vi "broadcast_ping.vi"() -> ()   [LabVIEW 2022 SP3]
uses:
  Library/dxl_x64_c.lvlib
panel:
  out "dynamixel_comm_result":string
  in  "dynamixel_id_list":string[][](table)=[[""], [""]]
  in  "device_name":string="COM1"
  out "protocol_version":dbl=2.0
  out "port_num":i32
  in  "baud_rate":i32=57600
  # "/*******************************************************************************\n* Copyright (c) 2016, ROBOTIS CO., LTD.\n* All rights reserved.\n*\n* Redistribution and use in source and binary forms, with or without\n* modification, are permitted provided that the following conditions are met:\n*\n* * Redistributions of source code must retain the above copyright notice, this\n*   list of conditions and the following disclaimer.\n*\n* * Redistributions in binary form must reproduce the above copyright notice,\n*   this list of conditions and the following disclaimer in the documentation\n*   and/or other materials provided with the distribution.\n*\n* * Neither the name of ROBOTIS nor the names of its\n*   contributors may be used to endorse or promote products derived from\n*   this software without specific prior written permission.\n*\n* THIS SOFTWARE IS PROVIDED BY THE COPYRIGHT HOLDERS AND CONTRIBUTORS \"AS IS\"\n* AND ANY EXPRESS OR IMPLIED WARRANTIES, INCLUDING, BUT NOT LIMITED TO, THE\n* IMPLIED WARRANTIES OF MERCHANTABILITY AND FITNESS FOR A PARTICULAR PURPOSE ARE\n* DISCLAIMED. IN NO EVENT SHALL THE COPYRIGHT HOLDER OR CONTRIBUTORS BE LIABLE\n* FOR ANY DIRECT, INDIRECT, INCIDENTAL, SPECIAL, EXEMPLARY, OR CONSEQUENTIAL\n* DAMAGES (INCLUDING, BUT NOT LIMITED TO, PROCUREMENT OF SUBSTITUTE GOODS OR\n* SERVICES; LOSS OF USE, DATA, OR PROFITS; OR BUSINESS INTERRUPTION) HOWEVER\n* CAUSED AND ON ANY THEORY OF LIABILITY, WHETHER IN CONTRACT, STRICT LIABILITY,\n* OR TORT (INCLUDING NEGLIGENCE OR OTHERWISE) ARISING IN ANY WAY OUT OF THE USE\n* OF THIS SOFTWARE, EVEN IF ADVISED OF THE POSSIBILITY OF SUCH DAMAGE.\n*******************************************************************************/\n\n/* Author: Ryu Woon Jung (Leon) */"
  # "Available Dynamixel model on this example : All models using Protocol 2.0\nThis example is designed for using Dynamixel PRO 54-200s, and an USB2DYNAMIXEL.\nTo use another Dynamixel model, such as X series, see their details in E-Manual(support.robotis.com) \n   and edit \"numeric control\"s seen left with \"Edit Text\" tool.\nBe sure that Dynamixel PRO properties are already set as %% ID : 1 / Baudnum : 1 (Baudrate : 57600)\n\n1. Run example by click above \"Run\" button (below \"Edit\" menu).\n2. You may see the ID list of connected Dynamixels."
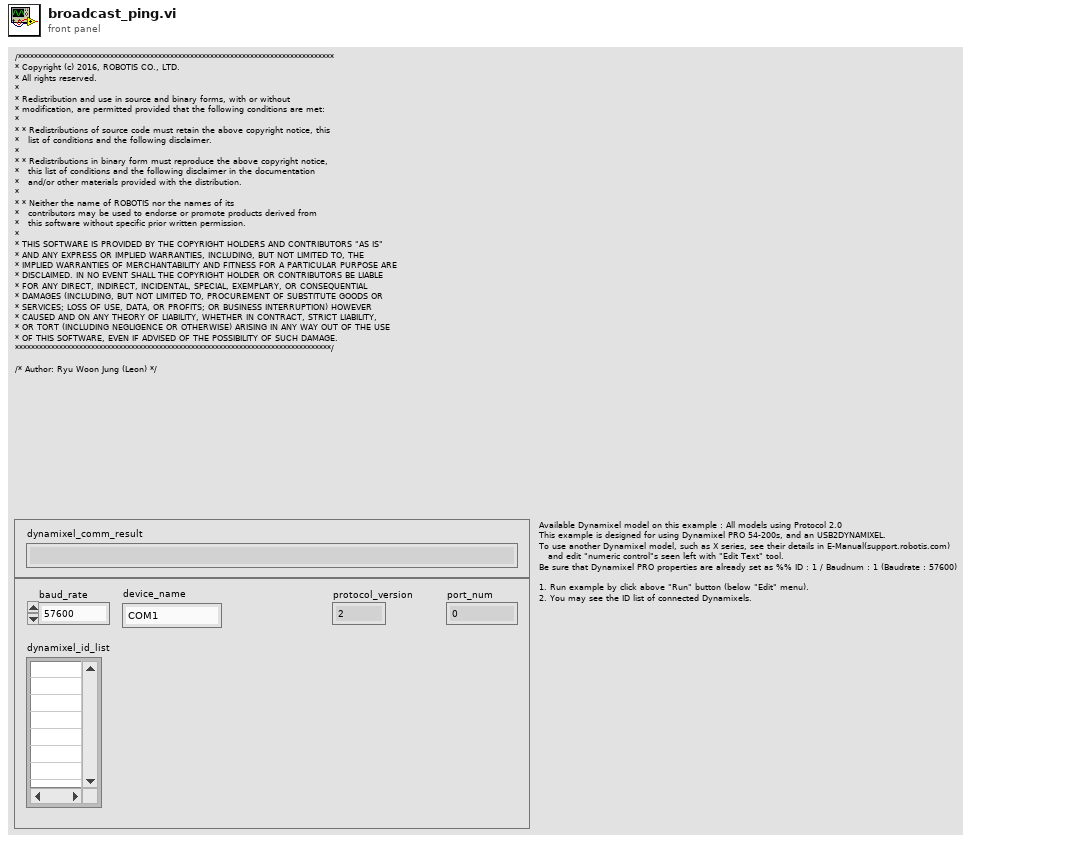
[diagram p1: front panel]
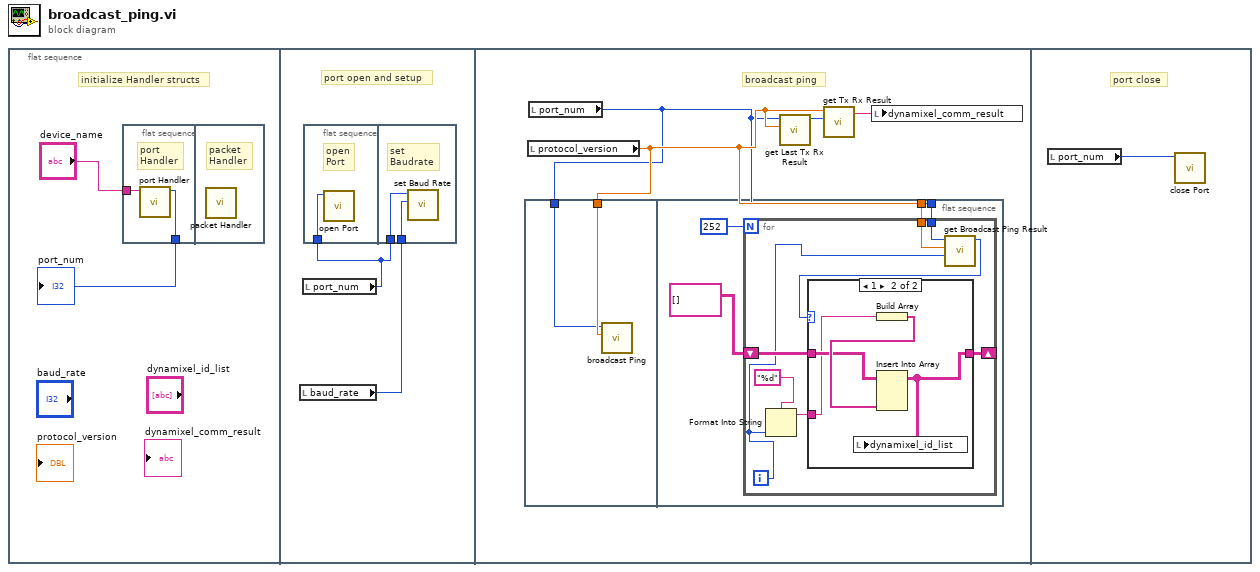
[diagram p0: block diagram]
diagram:
  n1 = flat-sequence {
    frame #0 {
      # "initialize Handler structs"
      n2 = flat-sequence {
        tunnel: [w4] -> w2
        tunnel: "device_name" -> [w3]
        frame #0 {
          # "port\nHandler"
          n3 = call "port Handler.vi"("port_name"=w3) -> ("function return"=w4:i32)  [unwired: 9 in, 1 out]
        }
        frame #1 {
          # "packet\nHandler"
          n4 = call "packet Handler.vi"() -> ()  [unwired: 11 in, 1 out]
        }
      }
      "port_num" <- w2
    }
    frame #1 {
      # "port open and setup"
      n5 = local read "baud_rate"() -> (w5:i32)
      n6 = local read "port_num"() -> (w6:i32)
      n7 = flat-sequence {
        tunnel: w6 -> [w7]
        tunnel: w6 -> [w9]
        tunnel: w5 -> [w8]
        frame #0 {
          # "open\nPort"
          n8 = call "open Port.vi"("port_num"=w7) -> ()  [unwired: 9 in, 2 out]
        }
        frame #1 {
          # "set\nBaudrate"
          n9 = call "set Baud Rate.vi"("baudrate"=w8, "port_num"=w9) -> ()  [unwired: 8 in, 2 out]
        }
      }
    }
    frame #2 {
      # "broadcast ping"
      n10 = flat-sequence {
        tunnel: w11 -> [w15]
        tunnel: w10 -> [w14]
        tunnel: w11 -> [w18]
        tunnel: w10 -> [w17]
        frame #0 {
          n11 = call "broadcast Ping.vi"("protocol_version"=w15, "port_num"=w14) -> ()  [unwired: 9 in, 1 out]
        }
        frame #1 {
          n12 = for {
            N: 252 -> [_]
            tunnel: w18 -> [w26]
            tunnel: w17 -> [w25]
            shift-right: [w23] -> _
            shift-left: string[][] [] -> [w24]
            i -> [w20]
            n13 = Format Into String(format string="%d", w20) -> (resulting string=w21:string)  [unwired: 2 in, 1 out]
            n14 = call "get Broadcast Ping Result.vi"("id"=w20, "protocol_version"=w26, "port_num"=w25) -> ("function return"=w27:u8)  [unwired: 7 in, 1 out]
            n15 = case shown="1" w27 {
              tunnel: w24 -> [w28 w31]
              tunnel: [w28 w29] -> w23
              tunnel: w21 -> [_ w30]
              frame 0, Default {
              }
              frame 1 {
                n16 = Build Array(w30) -> (w32:string[])
                n17 = Insert Into Array(array=w31, new element=w32) -> (w29:string[][])  [unwired: 2 in]
                n18 = local write "dynamixel_id_list"(w29) -> ()
              }
            }
          }
        }
      }
      n19 = local read "protocol_version"() -> (w11:dbl)
      n20 = local read "port_num"() -> (w10:i32)
      n21 = call "get Last Tx Rx Result.vi"("protocol_version"=w11, "port_num"=w10) -> ("function return"=w12:i32)  [unwired: 8 in, 1 out]
      n22 = call "get Tx Rx Result.vi"("result"=w12, "protocol_version"=w11) -> ("function return"=w13:string)  [unwired: 8 in, 1 out]
      n23 = local write "dynamixel_comm_result"(w13) -> ()
    }
    frame #3 {
      # "port close"
      n24 = local read "port_num"() -> (w33:i32)
      n25 = call "close Port.vi"("port_num"=w33) -> ()  [unwired: 10 in, 1 out]
    }
  }
